vi "test Parse Double.vi"() -> (0 "error out":errorcluster, 2 "pass?":bool)   [LabVIEW 2019, in "RESP3 Tests.lvlib"]
uses:
  RESP3 Tests.lvlib
  RESP3/RESP3 Parser/RESP3 Parser.lvclass
  RESP3/types/RESP3 Type.ctl
  RESP3/types/RESP3 data type attribute.vi
  RESP3/RESP3.lvlib
  RESP3/high-level/RESP3 Get Double.vi
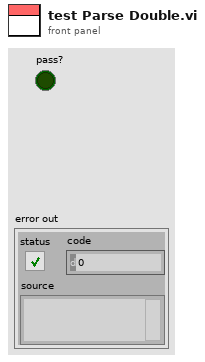
[diagram p1: front panel]
types:
  T1 = typedef "RESP3.lvlib/RESP3 Type.ctl" = enum8{"<0x00>", "<0x01>", "<0x02>", "<0x03>", "<0x04>", "<0x05>", "<0x06>", "<0x07>", "<0x08>", "<0x09>", "<0x0A>", "<0x0B>", "<0x0C>", "<0x0D>", "<0x0E>", "<0x0F>", "<0x10>", "<0x11>", "<0x12>", "<0x13>", "<0x14>", "<0x15>", "<0x16>", "<0x17>", "<0x18>", "<0x19>", "<0x1A>", "<0x1B>", "<0x1C>", "<0x1D>", "<0x1E>", "<0x1F>", "\" \"", "BLOB ERROR", "\"\"\"", "BOOLEAN", "BLOB", "MAP", "\"&\"", "\"'\"", "BIG NUMBER", "\")\"", "ARRAY", "STRING", "DOUBLE", "ERROR", "END", "\"/\"", "\"0\"", "\"1\"", "\"2\"", "\"3\"", "\"4\"", "\"5\"", "\"6\"", "\"7\"", "\"8\"", "\"9\"", "INTEGER", "STREAM", "\"<\"", "VERBATIM STRING", "PUSH", "\"?\"", "\"@\"", "\"A\"", "\"B\"", "\"C\"", "\"D\"", "\"E\"", "\"F\"", "\"G\"", "\"H\"", "\"I\"", "\"J\"", "\"K\"", "\"L\"", "\"M\"", "\"N\"", "\"O\"", "\"P\"", "\"Q\"", "\"R\"", "\"S\"", "\"T\"", "\"U\"", "\"V\"", "\"W\"", "\"X\"", "\"Y\"", "\"Z\"", "\"[\"", "\"\\\"", "\"]\"", "\"^\"", "NULL", "\"`\"", "\"a\"", "\"b\"", "\"c\"", "\"d\"", "\"e\"", "\"f\"", "\"g\"", "\"h\"", "\"i\"", "\"j\"", "\"k\"", "\"l\"", "\"m\"", "\"n\"", "\"o\"", "\"p\"", "\"q\"", "\"r\"", "\"s\"", "\"t\"", "\"u\"", "\"v\"", "\"w\"", "\"x\"", "\"y\"", "\"z\"", "\"{\"", "ATTRIBUTES", "\"}\"", "SET", "<0x7F>", "<0x80>", "<0x81>", "<0x82>", "<0x83>", "<0x84>", "<0x85>", "<0x86>", "<0x87>", "<0x88>", "<0x89>", "<0x8A>", "<0x8B>", "<0x8C>", "<0x8D>", "<0x8E>", "<0x8F>", "<0x90>", "<0x91>", "<0x92>", "<0x93>", "<0x94>", "<0x95>", "<0x96>", "<0x97>", "<0x98>", "<0x99>", "<0x9A>", "<0x9B>", "<0x9C>", "<0x9D>", "<0x9E>", "<0x9F>", "<0xA0>", "<0xA1>", "<0xA2>", "<0xA3>", "<0xA4>", "<0xA5>", "<0xA6>", "<0xA7>", "<0xA8>", "<0xA9>", "<0xAA>", "<0xAB>", "<0xAC>", "<0xAD>", "<0xAE>", "<0xAF>", "<0xB0>", "<0xB1>", "<0xB2>", "<0xB3>", "<0xB4>", "<0xB5>", "<0xB6>", "<0xB7>", "<0xB8>", "<0xB9>", "<0xBA>", "<0xBB>", "<0xBC>", "<0xBD>", "<0xBE>", "<0xBF>", "<0xC0>", "<0xC1>", "<0xC2>", "<0xC3>", "<0xC4>", "<0xC5>", "<0xC6>", "<0xC7>", "<0xC8>", "<0xC9>", "<0xCA>", "<0xCB>", "<0xCC>", "<0xCD>", "<0xCE>", "<0xCF>", "<0xD0>", "<0xD1>", "<0xD2>", "<0xD3>", "<0xD4>", "<0xD5>", "<0xD6>", "<0xD7>", "<0xD8>", "<0xD9>", "<0xDA>", "<0xDB>", "<0xDC>", "<0xDD>", "<0xDE>", "<0xDF>", "<0xE0>", "<0xE1>", "<0xE2>", "<0xE3>", "<0xE4>", "<0xE5>", "<0xE6>", "<0xE7>", "<0xE8>", "<0xE9>", "<0xEA>", "<0xEB>", "<0xEC>", "<0xED>", "<0xEE>", "<0xEF>", "<0xF0>", "<0xF1>", "<0xF2>", "<0xF3>", "<0xF4>", "<0xF5>", "<0xF6>", "<0xF7>", "<0xF8>", "<0xF9>", "<0xFA>", "<0xFB>", "<0xFC>", "<0xFD>", "<0xFE>"}
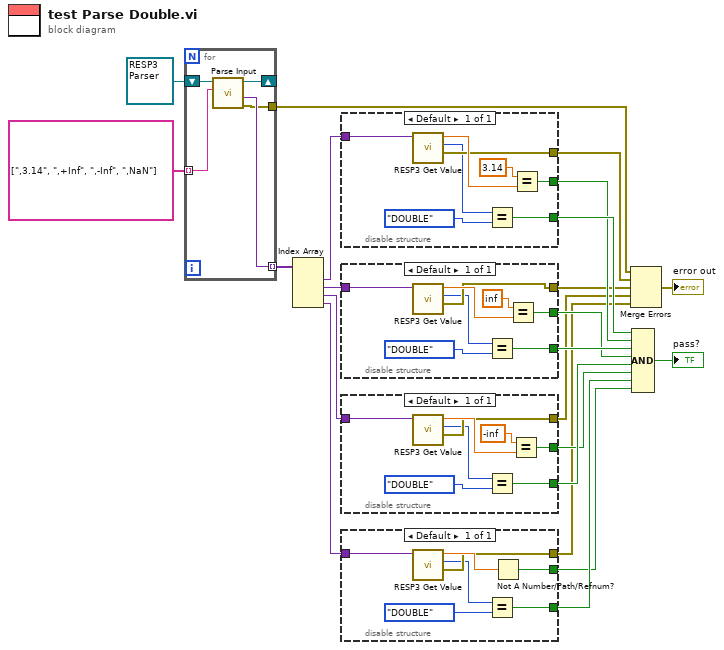
[diagram p0: block diagram]
diagram:
  n1 = for {
    shift-right: [w26] -> _
    shift-left: refnum<class "RESP3 Parser.lvclass"> refnum ("RESP3.lvlib:RESP3 Parser.lvclass") -> [w27]
    tunnel: string[] [",3.14", ",+Inf", ",-Inf", ",NaN"] -> [w25] mode=indexing
    tunnel: [w24] -> w17 mode=indexing
    tunnel: [w23] -> w1
    n2 = call-dynamic "Parse Input.vi"("input line"=w25, "RESP3 Parser in"=w27) -> ("error out"=w23:errorcluster, "RESP3 Value"=w24:variant, "RESP3 Parser out"=w26:refnum<class "RESP3 Parser.lvclass">)  [unwired: 5 in, 2 out]
  }
  n3 = Index Array(array=w17) -> (element #1=w15:variant, element #2=w14:variant, element #3=w13:variant, element #4=w12:variant)  [unwired: 4 in]
  n4 = disable-structure shown="Default" {
    disable-tunnel: [w34] -> w20
    disable-tunnel: [w32] -> w19
    disable-tunnel: w15 -> [w31]
    disable-tunnel: [w29] -> w16
    frame Enabled {
      n5 = call-poly "RESP3 Get Value.vi"("RESP3 Value in"=w31) -> ("error out"=w29:errorcluster, "actual RESP3 type"=w28:T1, "Number out"=w30:dbl)  [unwired: 8 in]
      n6 = Equal?(x=w28, y=RESP3_Type."DOUBLE") -> (x = y?=w34:bool)
      n7 = Equal?(x=3.14, y=w30) -> (x = y?=w32:bool)
    }
  }
  n8 = disable-structure shown="Default" {
    disable-tunnel: [w42] -> w11
    disable-tunnel: [w40] -> w10
    disable-tunnel: w14 -> [w39]
    disable-tunnel: [w37] -> w4
    frame Enabled {
      n9 = call-poly "RESP3 Get Value.vi"("RESP3 Value in"=w39) -> ("error out"=w37:errorcluster, "actual RESP3 type"=w36:T1, "Number out"=w38:dbl)  [unwired: 8 in]
      n10 = Equal?(x=w36, y=RESP3_Type."DOUBLE") -> (x = y?=w42:bool)
      n11 = Equal?(x=inf, y=w38) -> (x = y?=w40:bool)
    }
  }
  n12 = disable-structure shown="Default" {
    disable-tunnel: [w50] -> w9
    disable-tunnel: [w48] -> w8
    disable-tunnel: w13 -> [w47]
    disable-tunnel: [w45] -> w3
    frame Enabled {
      n13 = call-poly "RESP3 Get Value.vi"("RESP3 Value in"=w47) -> ("error out"=w45:errorcluster, "actual RESP3 type"=w44:T1, "Number out"=w46:dbl)  [unwired: 8 in]
      n14 = Equal?(x=w44, y=RESP3_Type."DOUBLE") -> (x = y?=w50:bool)
      n15 = Equal?(x=-inf, y=w46) -> (x = y?=w48:bool)
    }
  }
  n16 = disable-structure shown="Default" {
    disable-tunnel: [w57] -> w7
    disable-tunnel: [w56] -> w6
    disable-tunnel: w12 -> [w55]
    disable-tunnel: [w53] -> w2
    frame Enabled {
      n17 = call-poly "RESP3 Get Value.vi"("RESP3 Value in"=w55) -> ("error out"=w53:errorcluster, "actual RESP3 type"=w52:T1, "Number out"=w54:dbl)  [unwired: 8 in]
      n18 = Equal?(x=w52, y=RESP3_Type."DOUBLE") -> (x = y?=w57:bool)
      n19 = Not A Number/Path/Refnum?(number/path/refnum=w54) -> (NaN/Path/Refnum?=w56:bool)
    }
  }
  n20 = Merge Errors(w1, w16, w4, w3, w2) -> (→"error out":errorcluster)
  n21 = Compound Arithmetic op=AND(w20, w19, w11, w10, w9, w8, w7, w6) -> (→"pass?":bool)
